vi "Gyro.vi"   [LabVIEW 2016, in "Test.lvrbt"]
uses:
  Test.lvrbt
  <vilib>/NXT/Block Support/NXT_InputPort.ctl
  <vilib>/NXT/Hardware/Plugins/Tetrix DC Motor/TetrixDCMotorAddress.ctl
  <vilib>/NXT/Dual Mode Library/Waits/Wait_Num.vi
  <vilib>/NXT/NXTIO Xnodes/NXTIONodeSubVIs/TETRIX IO Move DC Motors.vi
  <vilib>/NXT/Dual Mode Library/Waits/Wait_EV3_Angle_Less.vi
  <vilib>/NXT/NXTIO Xnodes/NXTIONodeSubVIs/TETRIX IO Stop DC Motors.vi
  <vilib>/NXT/Dual Mode Library/Waits/Wait_EV3_Angle_Greater.vi
  <vilib>/NXT/NXTIO Xnodes/AddressXNode/NXTIOAddress.xnode
  <vilib>/NXT/NXTIO Xnodes/NXTIOXNode/NXTIO.xnode
  <vilib>/NXT/Subs/LVHSConnector.ctl
  <vilib>/NXT/LegoClasses/BrickReference/BrickReference.lvclass
types:
  T1 = typedef "NXT_InputPort.ctl" = u32
  T2 = typedef "LVHSConnector.ctl" = refnum<class "BrickReference.lvclass">
  T3 = typedef "TetrixDCMotorAddress.ctl" = i32
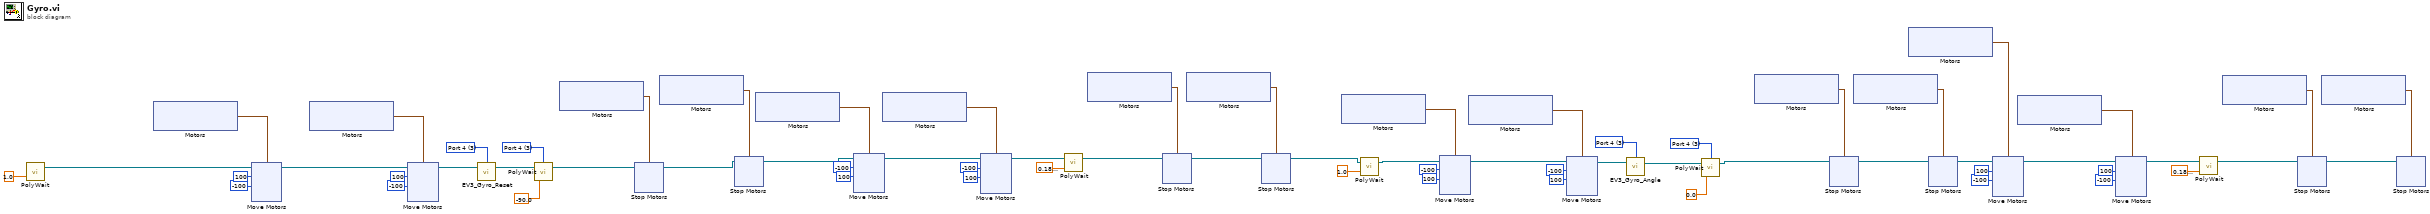
[diagram p0: block diagram]
diagram:
  w33 = T1 3 items=["Port 1", "Port 2", "Port 3", "Port 4"] ("Port (Port 1)")
  w34 = T1 3 items=["Port 1", "Port 2", "Port 3", "Port 4"] ("Port (Port 1)")
  w56 = T1 3 items=["Port 1", "Port 2", "Port 3", "Port 4"] ("Port (Port 1)")
  w65 = T1 3 items=["Port 1", "Port 2", "Port 3", "Port 4"] ("Port (Port 1)")
  n1 = call-poly <vilib>:"PolyWait.vi"("Time (1 sec)"=sgl 1.0) -> ("NXT/EV3"=w50:T2)  [unwired: 3 in]
  n2 = xnode "Motors"() -> ("Motor"=w54:cluster{"TetrixDCMotor":T3, "TetrixDCMotor":T3})
  n3 = xnode "Move Motors"("Power/Speed 2"=i8 -100, "Power/Speed 1"=i8 100, "Motors"=w54, "NXT/EV3"=w50) -> ("NXT/EV3"=w51:T2)
  n4 = xnode "Motors"() -> ("Motor"=w64:cluster{"TetrixDCMotor":T3, "TetrixDCMotor":T3})
  n5 = xnode "Move Motors"("Power/Speed 2"=i8 -100, "Power/Speed 1"=i8 100, "Motors"=w64, "NXT/EV3"=w51) -> ("NXT/EV3"=w59:T2)
  n6 = call <vilib>:"EV3_Gyro_Reset.vi"("NXT/EV3"=w59, "Port (Port 1)"=w65) -> ("NXT/EV3"=w58:T2)  [unwired: 2 in]
  n7 = call-poly <vilib>:"PolyWait.vi"("Degrees (180)"=sgl -90.0, "NXT/EV3"=w58, "Port (Port 1)"=w56) -> ("NXT/EV3"=w57:T2)  [unwired: 1 in]
  n8 = xnode "Motors"() -> ("Motor"=w60:cluster{"TetrixDCMotor":T3, "TetrixDCMotor":T3})
  n9 = xnode "Stop Motors"("Motors"=w60, "NXT/EV3"=w57) -> ("NXT/EV3"=w48:T2)
  n10 = xnode "Motors"() -> ("Motor"=w49:cluster{"TetrixDCMotor":T3, "TetrixDCMotor":T3})
  n11 = xnode "Stop Motors"("Motors"=w49, "NXT/EV3"=w48) -> ("NXT/EV3"=w22:T2)
  n12 = xnode "Motors"() -> ("Motor"=w29:cluster{"TetrixDCMotor":T3, "TetrixDCMotor":T3})
  n13 = xnode "Move Motors"("Power/Speed 2"=i8 100, "Power/Speed 1"=i8 -100, "Motors"=w29, "NXT/EV3"=w22) -> ("NXT/EV3"=w23:T2)
  n14 = xnode "Motors"() -> ("Motor"=w26:cluster{"TetrixDCMotor":T3, "TetrixDCMotor":T3})
  n15 = xnode "Move Motors"("Power/Speed 2"=i8 100, "Power/Speed 1"=i8 -100, "Motors"=w26, "NXT/EV3"=w23) -> ("NXT/EV3"=w17:T2)
  n16 = call-poly <vilib>:"PolyWait.vi"("Time (1 sec)"=sgl 0.18, "NXT/EV3"=w17) -> ("NXT/EV3"=w16:T2)  [unwired: 2 in]
  n17 = xnode "Motors"() -> ("Motor"=w21:cluster{"TetrixDCMotor":T3, "TetrixDCMotor":T3})
  n18 = xnode "Stop Motors"("Motors"=w21, "NXT/EV3"=w16) -> ("NXT/EV3"=w19:T2)
  n19 = xnode "Motors"() -> ("Motor"=w20:cluster{"TetrixDCMotor":T3, "TetrixDCMotor":T3})
  n20 = xnode "Stop Motors"("Motors"=w20, "NXT/EV3"=w19) -> ("NXT/EV3"=w15:T2)
  n21 = xnode "Motors"() -> ("Motor"=w47:cluster{"TetrixDCMotor":T3, "TetrixDCMotor":T3})
  n22 = call-poly <vilib>:"PolyWait.vi"("Time (1 sec)"=sgl 1.0, "NXT/EV3"=w15) -> ("NXT/EV3"=w41:T2)  [unwired: 2 in]
  n23 = xnode "Move Motors"("Power/Speed 2"=i8 100, "Power/Speed 1"=i8 -100, "Motors"=w47, "NXT/EV3"=w41) -> ("NXT/EV3"=w36:T2)
  n24 = xnode "Motors"() -> ("Motor"=w39:cluster{"TetrixDCMotor":T3, "TetrixDCMotor":T3})
  n25 = xnode "Move Motors"("Power/Speed 2"=i8 100, "Power/Speed 1"=i8 -100, "Motors"=w39, "NXT/EV3"=w36) -> ("NXT/EV3"=w35:T2)
  n26 = call <vilib>:"EV3_Gyro_Angle.vi"("NXT/EV3"=w35, "Port (Port 1)"=w34) -> ("NXT/EV3"=w31:T2)  [unwired: 1 in, 1 out]
  n27 = call-poly <vilib>:"PolyWait.vi"("Degrees (180)"=sgl 0.0, "NXT/EV3"=w31, "Port (Port 1)"=w33) -> ("NXT/EV3"=w30:T2)  [unwired: 1 in]
  n28 = xnode "Motors"() -> ("Motor"=w44:cluster{"TetrixDCMotor":T3, "TetrixDCMotor":T3})
  n29 = xnode "Stop Motors"("Motors"=w44, "NXT/EV3"=w30) -> ("NXT/EV3"=w42:T2)
  n30 = xnode "Motors"() -> ("Motor"=w43:cluster{"TetrixDCMotor":T3, "TetrixDCMotor":T3})
  n31 = xnode "Motors"() -> ("Motor"=w14:cluster{"TetrixDCMotor":T3, "TetrixDCMotor":T3})
  n32 = xnode "Stop Motors"("Motors"=w43, "NXT/EV3"=w42) -> ("NXT/EV3"=w1:T2)
  n33 = xnode "Move Motors"("Power/Speed 2"=i8 -100, "Power/Speed 1"=i8 100, "Motors"=w14, "NXT/EV3"=w1) -> ("NXT/EV3"=w8:T2)
  n34 = xnode "Motors"() -> ("Motor"=w11:cluster{"TetrixDCMotor":T3, "TetrixDCMotor":T3})
  n35 = xnode "Move Motors"("Power/Speed 2"=i8 -100, "Power/Speed 1"=i8 100, "Motors"=w11, "NXT/EV3"=w8) -> ("NXT/EV3"=w3:T2)
  n36 = call-poly <vilib>:"PolyWait.vi"("Time (1 sec)"=sgl 0.18, "NXT/EV3"=w3) -> ("NXT/EV3"=w2:T2)  [unwired: 2 in]
  n37 = xnode "Motors"() -> ("Motor"=w7:cluster{"TetrixDCMotor":T3, "TetrixDCMotor":T3})
  n38 = xnode "Stop Motors"("Motors"=w7, "NXT/EV3"=w2) -> ("NXT/EV3"=w5:T2)
  n39 = xnode "Motors"() -> ("Motor"=w6:cluster{"TetrixDCMotor":T3, "TetrixDCMotor":T3})
  n40 = xnode "Stop Motors"("Motors"=w6, "NXT/EV3"=w5) -> ()  [unwired: 1 out]
